vi "Read enemy_ball_possesion.vi"(8 "error in (no error)":errorcluster, 11 "Events in":refnum<class "Events.lvclass">) -> (0 "error out":errorcluster, 2 "enemy_ball_possesion":bool, 3 "Events out":refnum<class "Events.lvclass">)   [LabVIEW 2021, in "Events.lvclass"]
uses:
  Events.lvclass
  Events.lvclass/Events.ctl
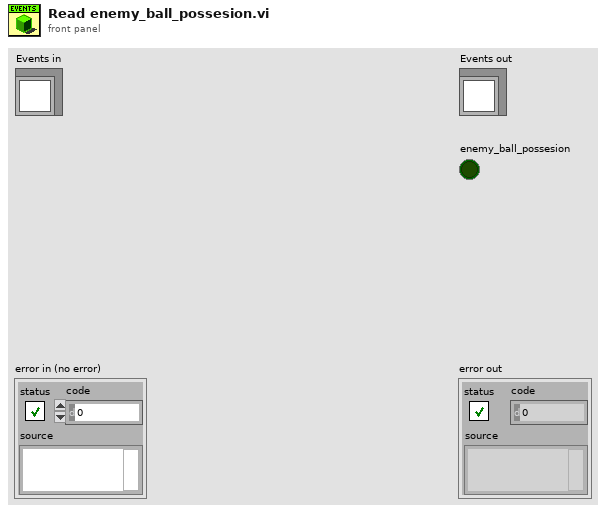
[diagram p1: front panel]
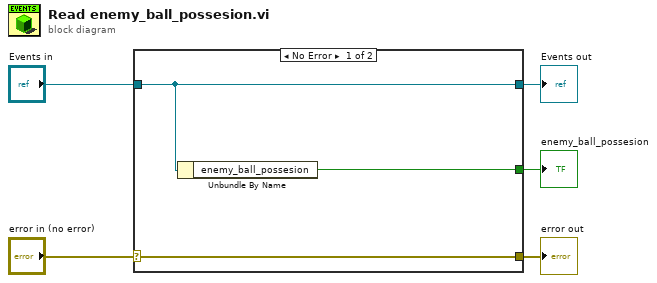
[diagram p0: block diagram]
diagram:
  n1 = case shown="No Error" "error in (no error)" {
    selector: "error in (no error)" -> [w8 w9]
    tunnel: [w8 w9] -> w4
    tunnel: [w7 w10] -> w2
    tunnel: "Events in" -> [w7 w10]
    tunnel: [w6 _] -> w1
    frame No Error {
      n2 = Unbundle By Name(w7) -> ("enemy_ball_possesion"=w6:bool)
    }
    frame Error {
    }
  }
  "error out" <- w4
  "Events out" <- w2
  "enemy_ball_possesion" <- w1
